vi "Set FM sweep.vi"(7 "Overall rep rate":dbl[unit]=50.0 min=0.0 format="%.2g", 8 "error in (no error)":errorcluster, 9 "# frequencies":u32=1 min=1 step=1, 10 "Start/stop frequencies":T1 {"stop" min=0.0 step=10000.0 format="%.2g"; "start" min=0.0 step=10000.0 format="%.2g"}, 11 "VISA resource name":refnum<visa-resource-name>) -> (0 "error out":errorcluster, 3 "VISA resource name out":refnum<visa-resource-name>)   [LabVIEW 2012]
doc: "Sets the function generator to sweep through three specified frequency ranges, at a given overall repetition rate. (Used for resonating the nuclei.) Takes advantage of the FM sweep mode of the function generator. Outputs on channel 1, so that we can use the trigger out to trigger the relays."
uses:
  <vilib>/imath/engines/lvmath2/RunTimeEngine/BuiltInFunctions/num_to_str/NIMS_num_to_str(GRowV,I32).vi
  <vilib>/imath/engines/lvmath/Plug In/_Char/NIMS_CH_String to Character Array.vi
  <vilib>/imath/engines/lvmath2/RunTimeEngine/BuiltInFunctions/strconcat/NIMS_strconcat.vi
  <vilib>/imath/engines/lvmath/Plug In/_Char/NIMS_CH_Character 2D to String 1D.vi
  <vilib>/imath/engines/lvmath/Plug In/_Char/NIMS_CH_String CV to Character 2D.vi
  <vilib>/imath/engines/lvmath2/RunTimeEngine/ErrorHandling/NIMS_Create Error From Enums.vi
  <vilib>/imath/engines/lvmath2/RunTimeEngine/RangeToken/NIMS_Range_R2 - Integer.vi
  <vilib>/imath/engines/lvmath2/RunTimeEngine/CommandStatement/MC_CommandStatement_break.vi
  <vilib>/imath/engines/lvmath2/RunTimeEngine/VariableToken/Read/NIMS_Get Elements - RV(_) - Check.vi
  <vilib>/imath/engines/lvmath2/RunTimeEngine/ReplaceToken/NIMS_Replace - V(S)=S.vi
  <vilib>/imath/engines/lvmath2/RunTimeEngine/ReplaceToken/NIMS_Replace - Check Linear.vi
  <vilib>/imath/engines/lvmath2/RunTimeEngine/ReplaceToken/NIMS_Replace - Size Check _(_)=S.vi
  <vilib>/imathl/engines/lvmath/Functions/Error Handling/Create Error.vi
  <vilib>/imath/engines/lvmath2/RunTimeEngine/BuiltInFunctions/sprintf/NIMS_sprintf(Str,RM).vi
  <vilib>/imath/engines/lvmath2/RunTimeSupport/NIMS_Get Row Vector_w Error - Matrix.vi
  <vilib>/imath/engines/lvmath/Plug In/_Char/NIMS_CH_Character RV to String.vi
  <vilib>/imath/engines/lvmath2/RunTimeEngine/NodeEndStatement/NIMS_NodeEndStatement_Output.vi
  <vilib>/imath/engines/lvmath2/RunTimeEngine/ErrorHandling/NIMS_Finalize Error.vi
  <vilib>/imath/engines/lvmath/Plug In/_Char/NIMS_CH_character datatype.ctl
  FG FM sweep start stop control.ctl
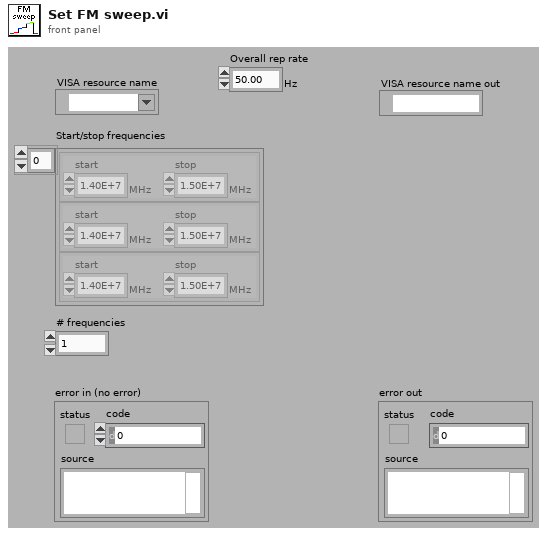
[diagram p1: front panel]
types:
  T1 = typedef "FG FM sweep start stop control.ctl" = cluster{"start":dbl[unit], "stop":dbl[unit]}[]
  T2 = typedef "NIMS_CH_character datatype.ctl" = cluster{"Numeric":u8}
  T3 = typedef "Semaphore RefNum" = refnum<k1>
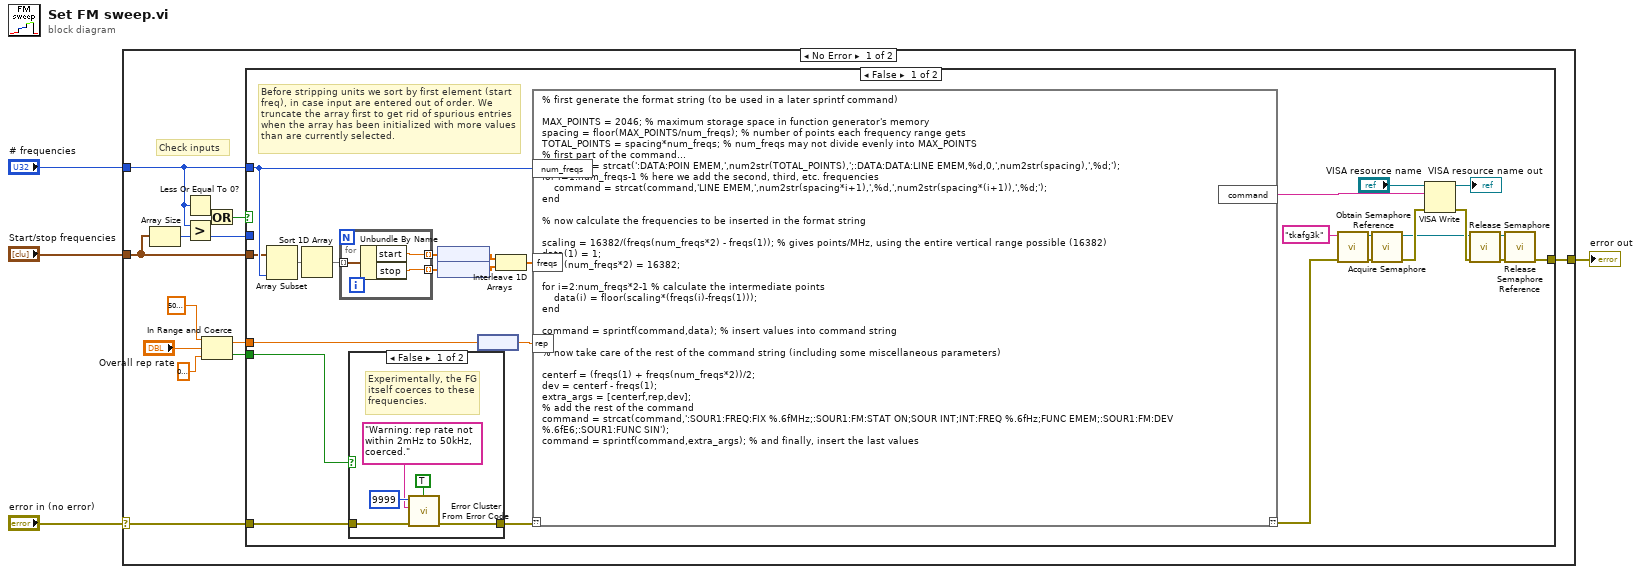
[diagram p0: block diagram]
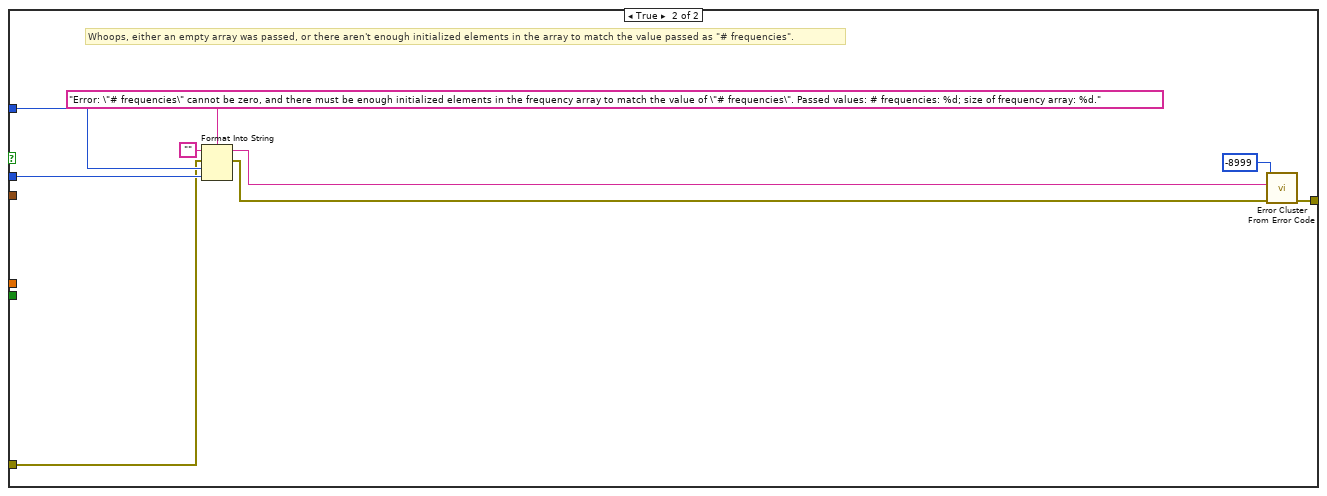
[diagram p3: hidden frame]
diagram:
  n1 = case shown="No Error" "error in (no error)" {
    selector: "error in (no error)" -> [w16 w456]
    tunnel: [w17 w456] -> w4
    tunnel: "Start/stop frequencies" -> [w5 _]
    tunnel: "# frequencies" -> [w15 _]
    frame No Error {
      # "Check inputs"
      n2 = Array Size(array=w5) -> (size(s)=w11:i32)
      n3 = Less Or Equal To 0?(x=w15) -> (x <= 0?=w14:bool)
      n4 = Greater?(x=w15, y=w11) -> (0:w13:bool)
      n5 = In Range and Coerce(upper limit=dbl[unit] 50000.0, x="Overall rep rate", lower limit=dbl[unit] 0.002 ("y")) -> (coerced(x)=w7:dbl[unit], In Range?=w8:bool)
      n6 = Or(x=w14, y=w13) -> (x .or. y?=w12:bool)
      n7 = case shown="False" w12 {
        tunnel: [w37 w454] -> w17
        tunnel: w16 -> [w25 w448]
        tunnel: w5 -> [w20 _]
        tunnel: w15 -> [w21 w451]
        tunnel: w11 -> [_ w450]
        tunnel: w7 -> [w23 _]
        tunnel: w8 -> [w22 _]
        frame False {
          # "Before stripping units we sort by first element (start freq), in case input are entered out of order. We truncate the array first to get rid of spurious entries when the array has been initialized with more values than are currently selected."
          n8 = Array Subset(array=w20, length=w21) -> (w19:T1)  [unwired: 1 in]
          n9 = Sort 1D Array(array=w19) -> (sorted array=w18:T1)
          n10 = for {
            tunnel: w18 -> [w446] mode=indexing
            tunnel: [w445] -> w34 mode=indexing
            tunnel: [w444] -> w35 mode=indexing
            n11 = Unbundle By Name(w446) -> ("start"=w445:dbl[unit], "stop"=w444:dbl[unit])
          }
          n12 = case shown="False" w22 {
            tunnel: w25 -> [w49 w50]
            tunnel: [w47 w50] -> w24
            frame False {
              # "Experimentally, the FG itself coerces to these frequencies."
              n13 = call <vilib>:"Error Cluster From Error Code.vi"("is warning? (False)"=TRUE, "error in (no error)"=w49, "error message (\"\")"="Warning: rep rate not within 2mHz to 50kHz, coerced." ("error message (\"\")"), "error code (0)"=9999) -> ("error out"=w47:errorcluster)  [unwired: 1 in, 4 out]
            }
            frame True {
            }
          }
          n14 = node(w34) -> (w33:dbl[])
          n15 = node(w35) -> (w32:dbl[])
          n16 = node(w23) -> (w30:dbl)
          n17 = Interleave 1D Arrays(w33, w32) -> (w31:dbl[])
          n18 = mathscript code="% first generate the format string (to be used in a later sprintf command)\n\nMAX_POINTS = 2046; % maximum storage space in function generator's memory\nspacing = floor(MAX_POINTS/num_freqs); % number of points each frequency range gets\nTOTAL_POINTS = spacing*num_freqs; % num_freqs may not divide evenly into MAX_POINTS\n% first part of the command...\ncommand = strcat(':DATA:POIN EMEM,',num2str(TOTAL_POINTS),';:DATA:DATA:LINE EMEM,%d,0,',num2str(spacing),',%d;');\nfor i=1:num_freqs-1 % here we add the second, third, etc. frequencies\n    command = strcat(command,'LINE EMEM,',num2str(spacing*i+1),',%d,',num2str(spacing*(i+1)),',%d;');\nend\n\n% now calculate the frequencies to be inserted in the format string\n\nscaling = 16382/(freqs(num_freqs*2) - freqs(1)); % gives points/MHz, using the entire vertical range possible (16382)\ndata(1) = 1;\ndata(num_freqs*2) = 16382;\n\nfor i=2:num_freqs*2-1 % calculate the intermediate points\n    data(i) = floor(scaling*(freqs(i)-freqs(1)));\nend\n\ncommand = sprintf(command,data); % insert values into command string\n\n% now take care of the rest of the command string (including some miscellaneous parameters)\n\ncenterf = (freqs(1) + freqs(num_freqs*2))/2;\ndev = centerf - freqs(1);\nextra_args = [centerf,rep,dev];\n% add the rest of the command\ncommand = strcat(command,':SOUR1:FREQ:FIX %.6fMHz;:SOUR1:FM:STAT ON;SOUR INT;INT:FREQ %.6fHz;FUNC EMEM;:SOUR1:FM:DEV %.6fE6;:SOUR1:FUNC SIN');\ncommand = sprintf(command,extra_args); % and finally, insert the last values"("??"=w24, "num_freqs"=w21, "freqs"=w31, "rep"=w30) -> ("??"=w28:errorcluster, "command"=w29:string)
          n19 = call <vilib>:"Obtain Semaphore Reference.vi"("error in (no error)"=w28, "name (unnamed)"="tkafg3k") -> ("error out"=w43:errorcluster, "semaphore"=w44:T3)  [unwired: 1 in, 3 out]
          n20 = call <vilib>:"Acquire Semaphore.vi"("error in (no error)"=w43, "semaphore"=w44) -> ("error out"=w42:errorcluster, "semaphore out"=w38:T3)  [unwired: 1 in, 3 out]
          n21 = VISA Write(VISA resource name="VISA resource name", write buffer=w29, error in (no error)=w42) -> (VISA resource name out=→"VISA resource name out":refnum<visa-resource-name>, error out=w39:errorcluster)  [unwired: 1 out]
          n22 = call <vilib>:"Release Semaphore.vi"("error in (no error)"=w39, "semaphore"=w38) -> ("error out"=w41:errorcluster, "semaphore out"=w40:T3)  [unwired: 4 out]
          n23 = call <vilib>:"Release Semaphore Reference.vi"("error in (no error)"=w41, "semaphore"=w40) -> ("error out"=w37:errorcluster)  [unwired: 9 out]
        }
        frame True {
          # "Whoops, either an empty array was passed, or there aren't enough initialized elements in the array to match the value passed as \"# frequencies\"."
          n24 = Format Into String(format string="Error: \"# frequencies\" cannot be zero, and there must be enough initialized elements in the frequency array to match the value of \"# frequencies\". Passed values: # frequencies: %d; size of frequency array: %d." ("error message (\"\")"), initial string="", error in=w448, w451, w450) -> (resulting string=w449:string, error out=w447:errorcluster)
          n25 = call <vilib>:"Error Cluster From Error Code.vi"("error in (no error)"=w447, "error message (\"\")"=w449, "error code (0)"=-8999) -> ("error out"=w454:errorcluster)  [unwired: 1 in, 5 out]
        }
      }
    }
    frame Error {
    }
  }
  "error out" <- w4
